vi "Save Document.vi"(8 "error in (no error)":errorcluster, 11 "Document in":refnum<class "npoiDocument.lvclass">) -> (0 "error out":errorcluster, 3 "Document out":refnum<class "npoiDocument.lvclass">)   [LabVIEW 2017, in "NPOI_Document.lvlib" / "npoiDocument.lvclass"]
doc: "Saves the <b>Document in</b> to the <b>Document Path</b> location given in the create or open method. Use get document path to retrieve the saved file location.\n\nNotes:\n - If <b>Document Path</b> is empty or is <Not A Path> or is a directory, the VI saves the document at a generated file path into the temporary directory."
uses:
  npoiDocument.lvclass
  npoiDocument.lvclass/npoiDocument.ctl
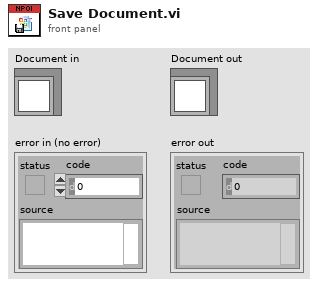
[diagram p1: front panel]
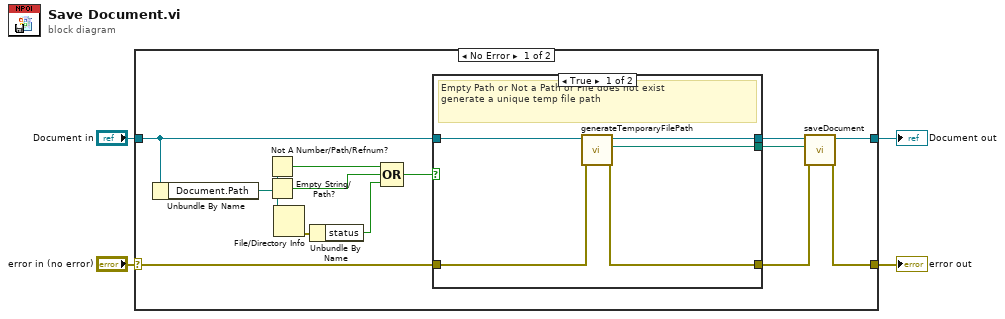
[diagram p0: block diagram]
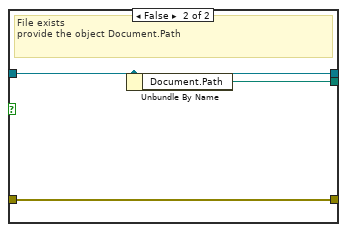
[diagram p2: hidden frame]
diagram:
  n1 = case shown="No Error" "error in (no error)" {
    selector: "error in (no error)" -> [w11 w27]
    tunnel: [w16 w27] -> w3
    tunnel: [w17 w26] -> w1
    tunnel: "Document in" -> [w12 w26]
    frame No Error {
      n2 = Unbundle By Name(w12) -> ("Document.Path"=w8:path)
      n3 = Not A Number/Path/Refnum?(number/path/refnum=w8) -> (NaN/Path/Refnum?=w14:bool)
      n4 = Empty String/Path?(string/path=w8) -> (empty?=w15:bool)
      n5 = File/Directory Info(path=w8) -> (error out=w7:errorcluster)  [unwired: 1 in, 6 out]
      n6 = Unbundle By Name(w7) -> ("status"=w6:bool)
      n7 = Compound Arithmetic op=OR(w14, w15, w6) -> (w13:bool)
      n8 = case shown="True" w13 {
        tunnel: w12 -> [w22 w24]
        tunnel: w11 -> [w20 w25]
        tunnel: [w21 w24] -> w10
        tunnel: [w19 w25] -> w9
        tunnel: [w18 w23] -> w5
        frame True {
          # "Empty Path or Not a Path or File does not exist\ngenerate a unique temp file path"
          n9 = call "generateTemporaryFilePath.vi"("error in (no error)"=w20, "npoiDocument in"=w22) -> ("error out"=w19:errorcluster, "Unique Temporary File Path"=w18:path, "npoiDocument out"=w21:refnum<class "npoiDocument.lvclass">)  [unwired: 7 in]
        }
        frame False {
          # "File exists\nprovide the object Document.Path"
          n10 = Unbundle By Name(w24) -> ("Document.Path"=w23:path)
        }
      }
      n11 = call-dynamic "saveDocument.vi"("error in (no error)"=w9, "Document Path"=w5, "npoiDocument in"=w10) -> ("error out"=w16:errorcluster, "npoiDocument out"=w17:refnum<class "npoiDocument.lvclass">)  [unwired: 7 in]
    }
    frame Error {
    }
  }
  "error out" <- w3
  "Document out" <- w1
